vi "Obtain Session.vi"(0 "Session  Name ()":string, 11 "error in (no error)":errorcluster) -> (4 "Session Handle":T1, 15 "error out":errorcluster)   [LabVIEW 2015, in "SLSC Switch.lvlib" / "SLSC Session.lvclass"]
doc: "This function initializes the measurement\n\nPass the function a name to obtain an active measurement handle"
uses:
  SLSC Session.lvclass
  Typedefs/Session Handle.ctl
  SLSC Session.lvclass/SLSC Session.ctl
  <userlib>/_Session Fwk/Session - Root.lvclass
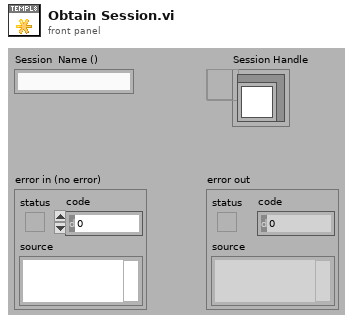
[diagram p1: front panel]
types:
  T1 = typedef "SLSC Switch.lvlib/SLSC Session.lvclass/Session Handle.ctl" = refnum<data-value>
  T2 = typedef "Session - Root.lvclass/Session Handle.ctl" = refnum<data-value>
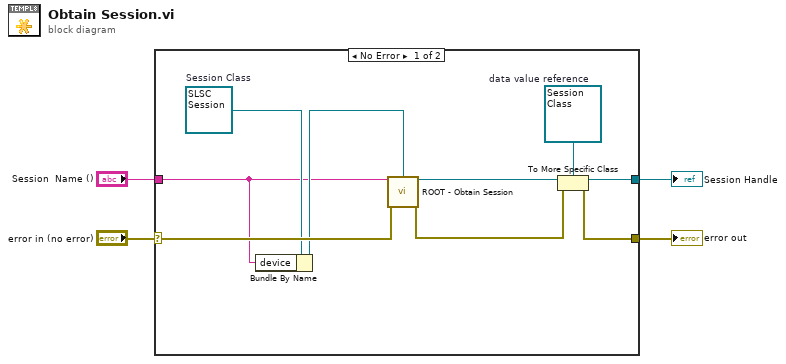
[diagram p0: block diagram]
diagram:
  n1 = case shown="No Error" "error in (no error)" {
    selector: "error in (no error)" -> [w13 w14]
    tunnel: [w10 w14] -> w3
    tunnel: [w12 _] -> w1
    tunnel: "Session  Name ()" -> [w5 _]
    frame No Error {
      w6 = refnum<data-value> refnum  # data value reference
      w7 = refnum<class "SLSC Session.lvclass"> refnum  # Session Class
      n2 = Bundle By Name(cluster=w7, "device"=w5) -> (w8:refnum<class "SLSC Session.lvclass">)
      n3 = call <userlib>:"ROOT - Obtain Session.vi"("Session Name ()"=w5, "OBJ - Session"=w8, "error in (no error)"=w13) -> ("Session Handle"=w9:T2, "error out"=w11:errorcluster)  [unwired: 10 in, 1 out]
      n4 = To More Specific Class(target class=w6, reference=w9, error in=w11) -> (specific class reference=w12:refnum<data-value>, error out=w10:errorcluster)
    }
    frame Error {
    }
  }
  "error out" <- w3
  "Session Handle" <- w1
